vi "L2R.vi"() -> ()   [LabVIEW 2022 SP3]
uses:
  <vilib>/regexp/Match Regular Expression.xnode
panel:
  in  "SET_scale":dbl=1.0 caption="scaling:" min=0.01 max=200.0 step=0.1
  in  "SET_rotate":bool
  in  "SET_term_z_offs":dbl=20.0 caption="terminal z \noffset:"
  in  "SET_term_moc":u16(ring) caption="terminal\nmovement:" items=["NONE", "INSIDE", "-X", "-Y", "Z ONLY"]
  in  "SET_x_offs":dbl caption="X offset:"
  in  "SET_y_offs":dbl caption="Y offset:"
  out "OUT_choice":bool
  out "OUT_file_num":i32 caption="split files created"
  out "CONV_splitting":bool caption="FILE SPLITTING"
  out "OUT_comm_lines":i32 caption="command lines found"
  in  "SET_max_lines":i32=2000 caption="max. file lines"
  in  "SET_tool_angl":bool caption="tool \nangulation:"
  out "FILE_name_old":string caption="old\nfilename:"
  in  "FILE_name_new":string caption="new \nfilename:"
  in  "SET_zone":i32=10 caption="zone:"
  in  "SET_tool":string="tool0" caption="tool:"
  in  "SET_movtype":u16(ring) caption="movement \ntype:" items=["LINEAR", "JOINT"]
  out "ERR_write_file":errorcluster
  out "OUT_rapid":string caption="RAPID string"
  out "CONV_running":bool caption="CONVERSION RUNNING"
  out "ERR_read_file":errorcluster caption="read file error"
  in  "FILE_path":path caption="file path:\n(dialog)"
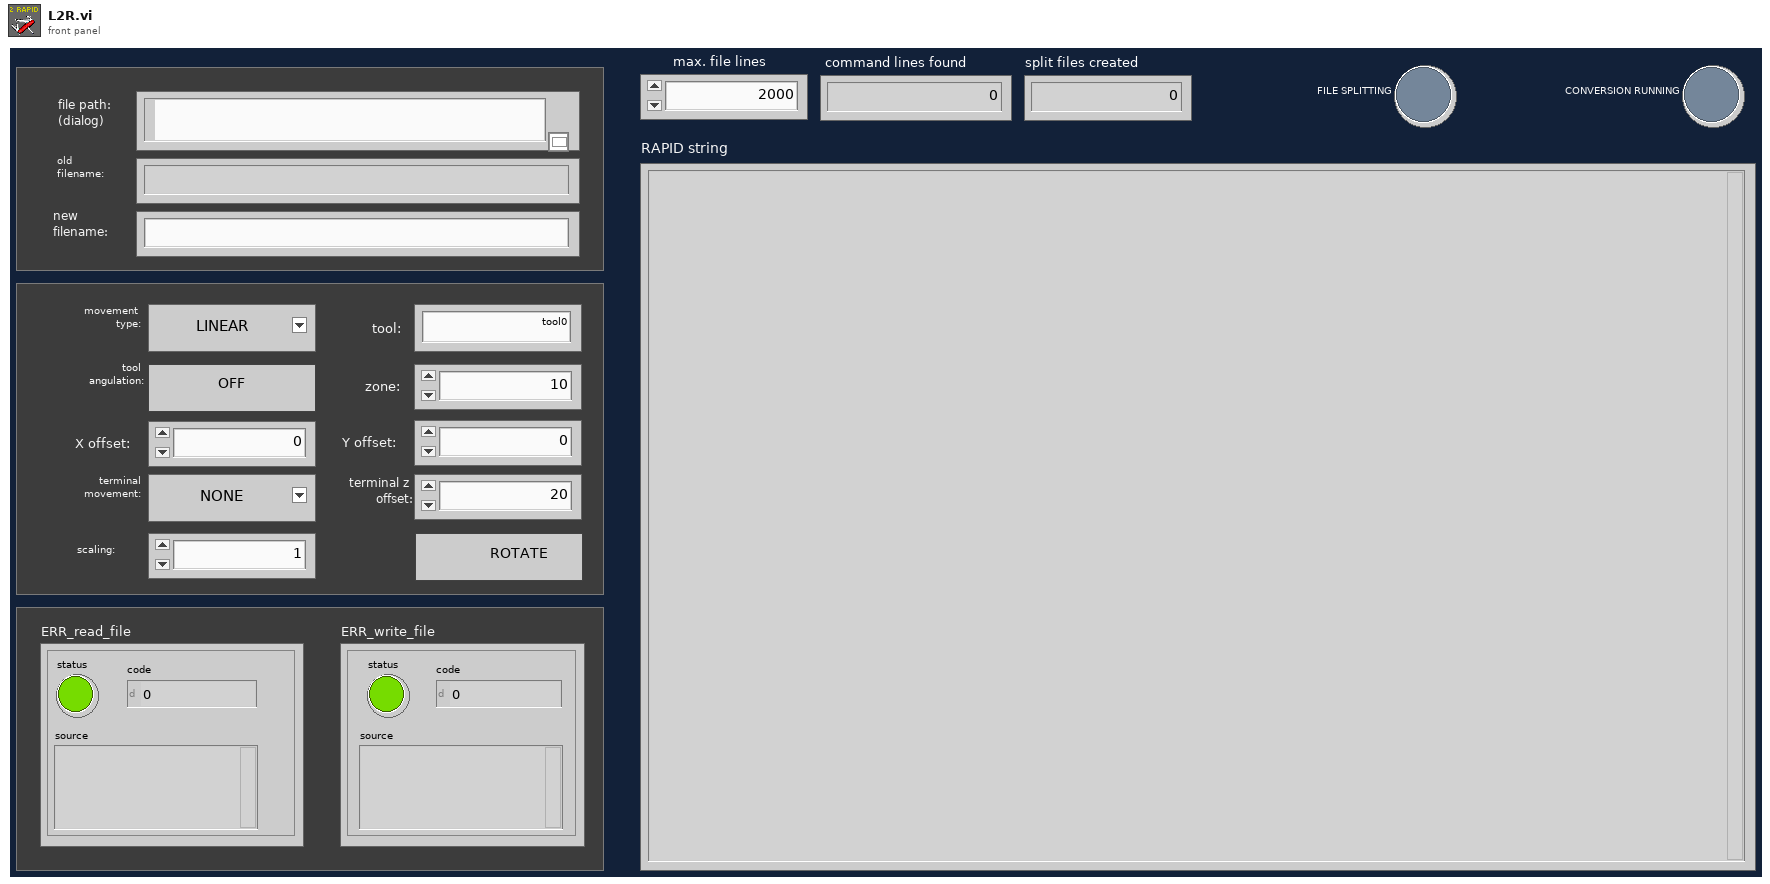
[diagram p1: front panel]
types:
  T1 = enum16{"open", "replace", "create", "open or create", "replace or create", "replace or create with confirmation"}
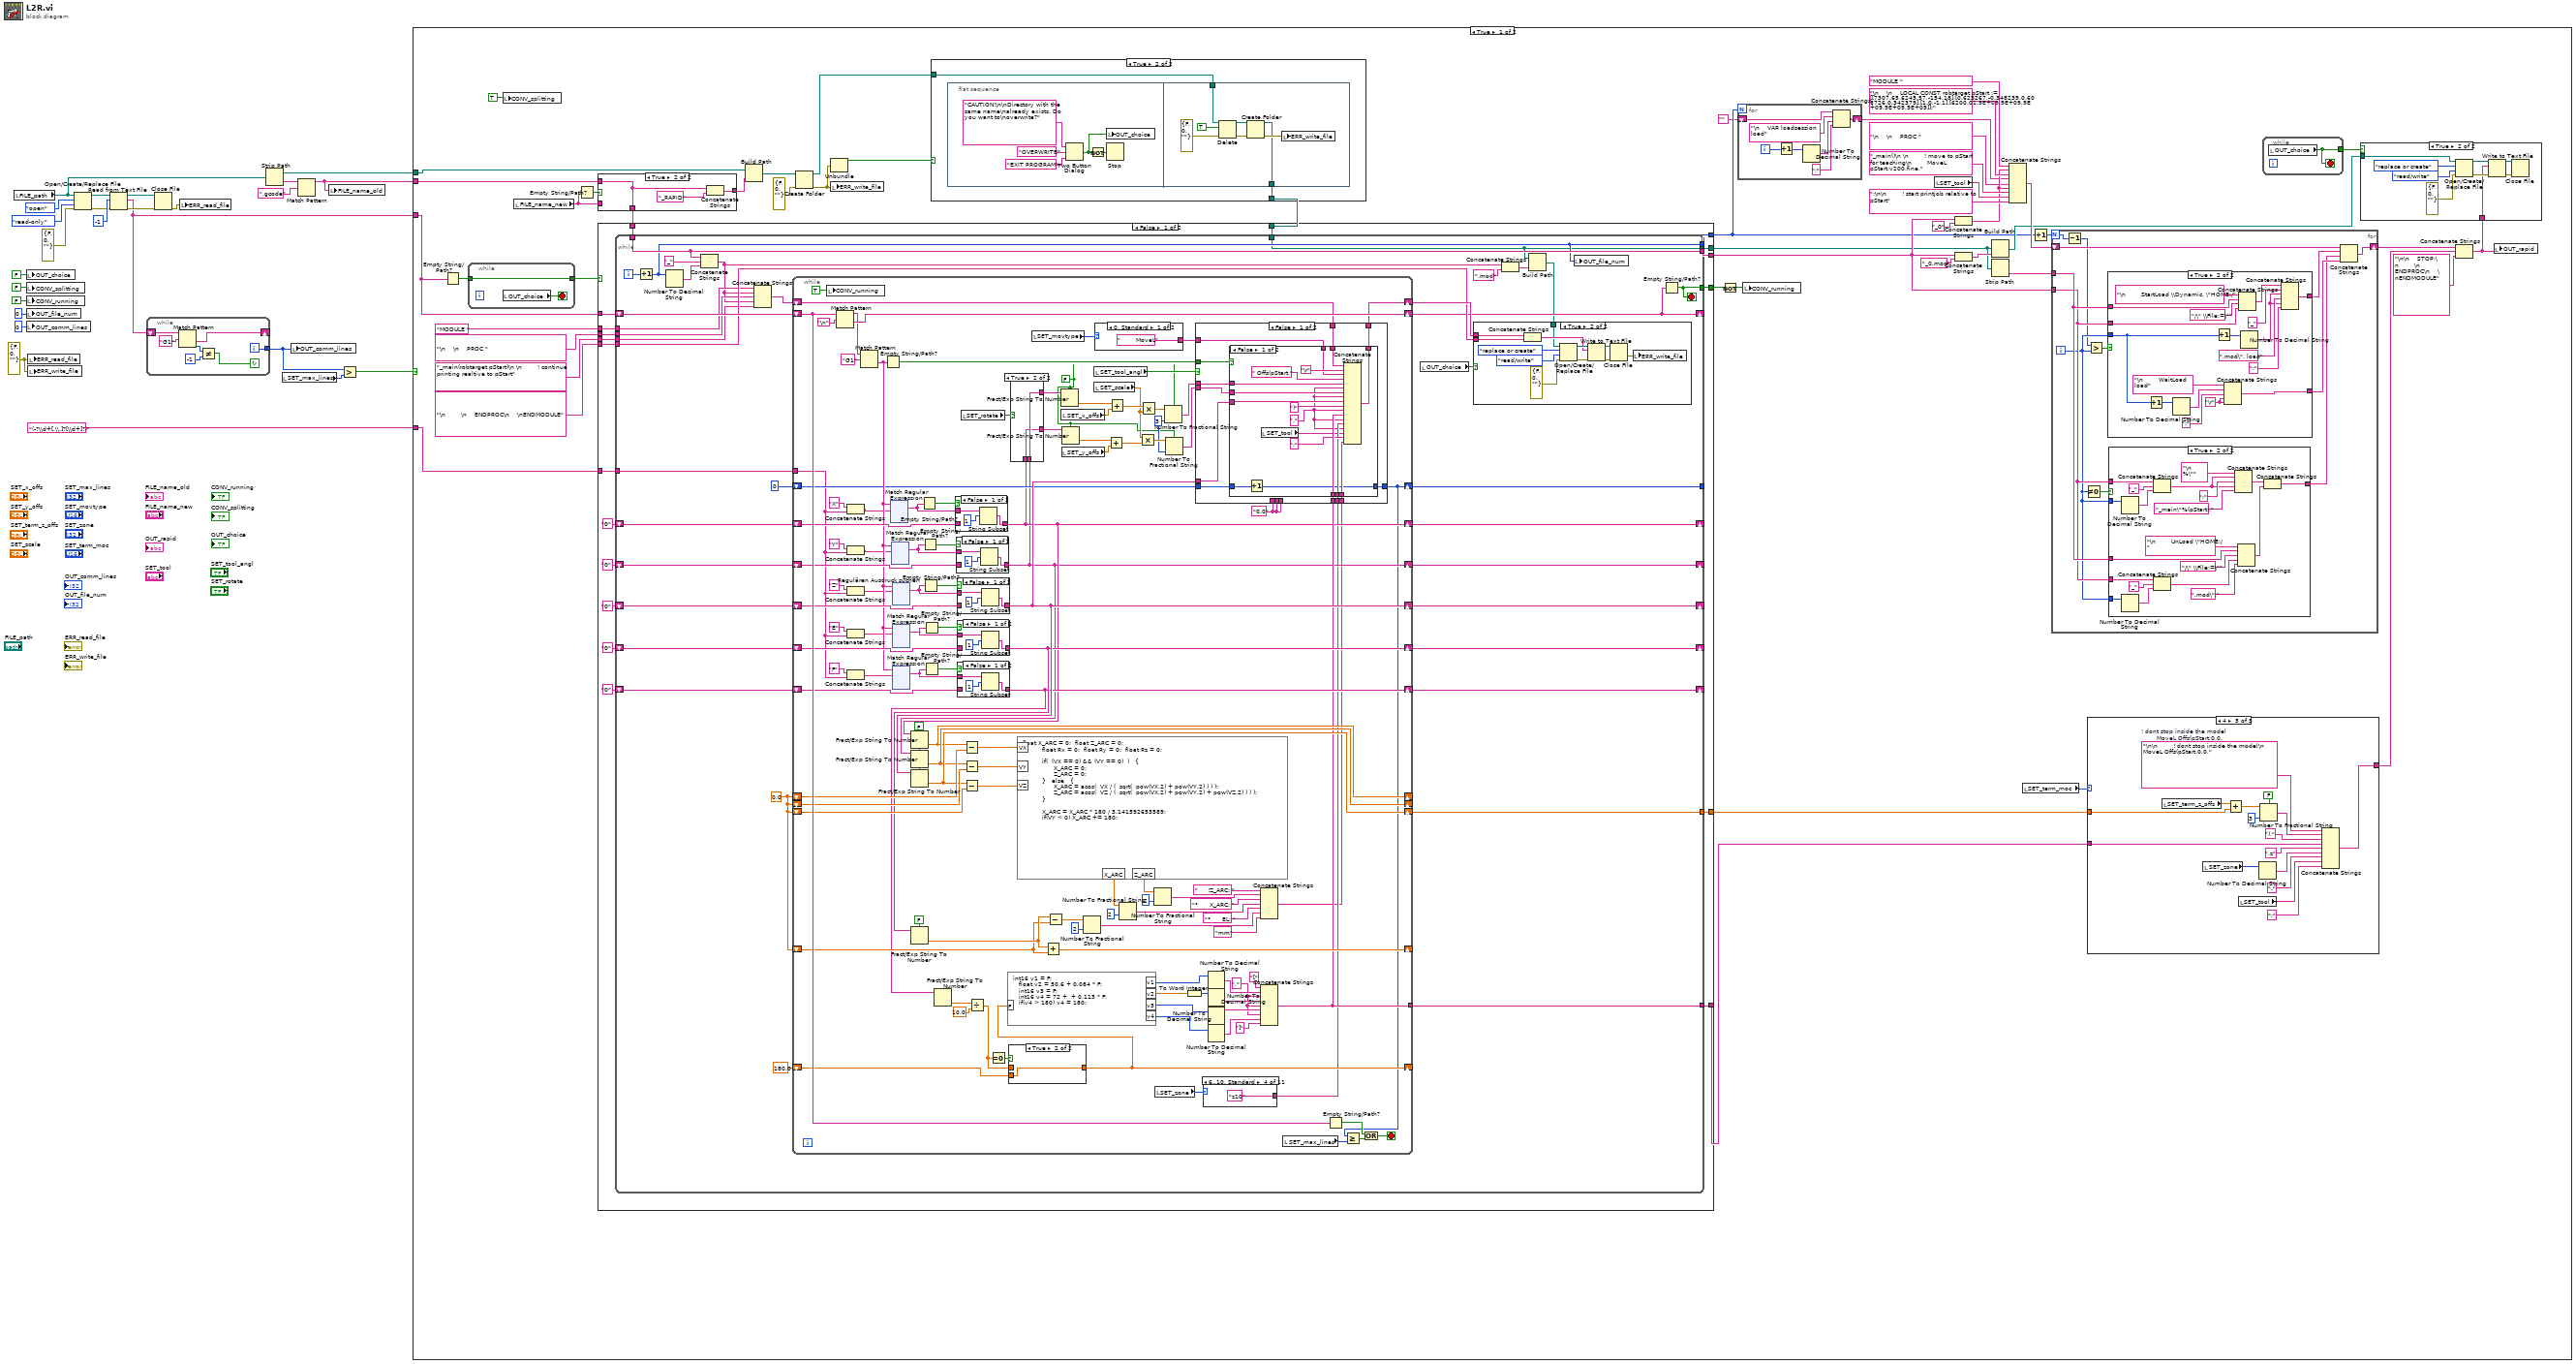
[diagram p0: block diagram]
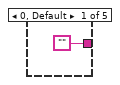
[diagram p2: hidden frame]
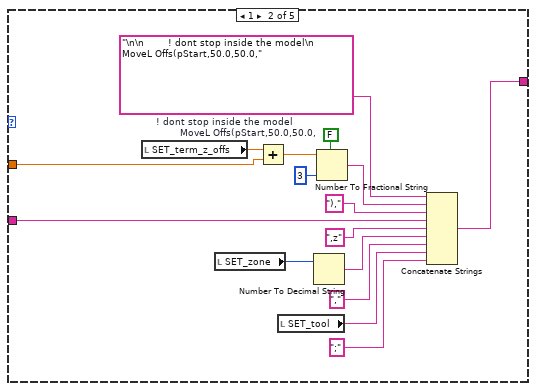
[diagram p3: hidden frame]
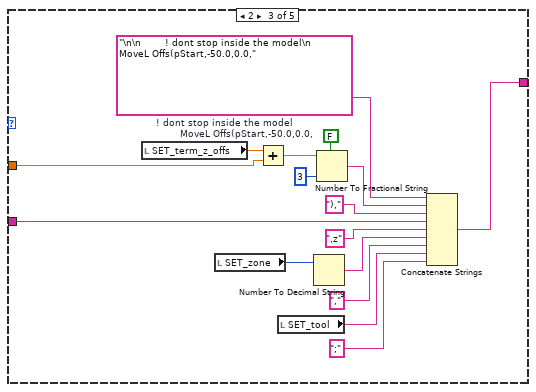
[diagram p4: hidden frame]
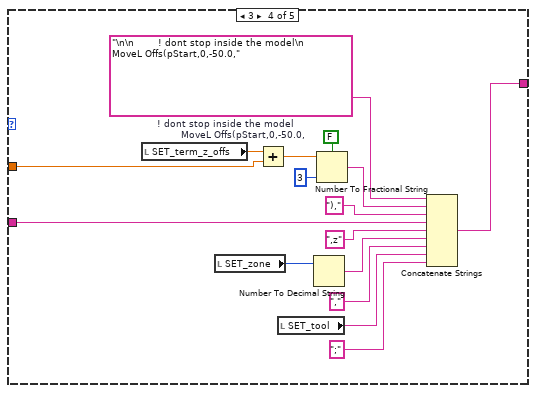
[diagram p5: hidden frame]
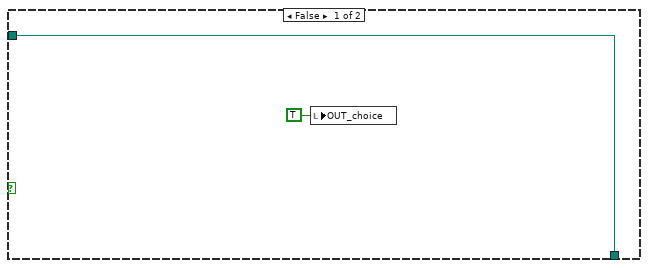
[diagram p7: hidden frame]
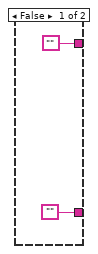
[diagram p8: hidden frame]
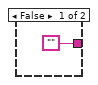
[diagram p9: hidden frame]
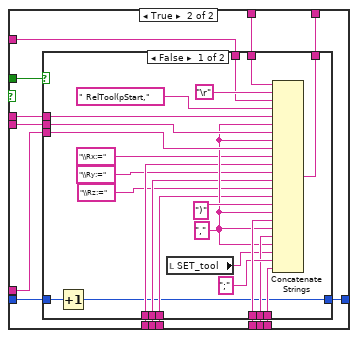
[diagram p15: hidden frame]
diagram:
  w6 = errorcluster {"status"=FALSE, "code"=0, "source"=""} ("ERR_write_file")
  n1 = local read "FILE_path"() -> (w10:path)
  n2 = local write "OUT_choice"(FALSE ("running")) -> ()
  n3 = local write "CONV_splitting"(FALSE ("running")) -> ()
  n4 = local write "CONV_running"(FALSE ("running")) -> ()
  n5 = local write "OUT_file_num"(0 ("OUT_file_num")) -> ()
  n6 = local write "OUT_comm_lines"(0 ("OUT_file_num")) -> ()
  n7 = local write "ERR_read_file"(w6) -> ()
  n8 = local write "ERR_write_file"(w6) -> ()
  n9 = Open/Create/Replace File(file path (use dialog)=w10, error in=errorcluster {"status"=FALSE, "code"=0, "source"=""}, operation (0:open)=T1."open", access (0:read/write)=enum16{"read/write", "read-only", "write-only"}."read-only") -> (refnum out=w21:refnum<file>, error out=w20:errorcluster)  [unwired: 2 in, 1 out]
  n10 = Read from Text File(file (use dialog)=w21, count=-1, error in=w20) -> (refnum out=w19:refnum<file>, text=w2:string, error out=w18:errorcluster)  [unwired: 1 in, 1 out]
  n11 = while {
    shift-right: [w30] -> _
    shift-left: w2 -> [w32]
    tunnel: [w26] -> w8
    i -> [w26]
    stop <- w27 continue-if-true
    n12 = Match Pattern(string=w32, regular expression="G1") -> (after substring=w30:string, offset past match=w29:i32)  [unwired: 1 in, 2 out]
    n13 = Not Equal?(x=w29, y=-1) -> (x != y?=w27:bool)
  }
  n14 = Close File(refnum=w19, error in=w18) -> (error out=w11:errorcluster)  [unwired: 1 out]
  n15 = local write "ERR_read_file"(w11) -> ()
  n16 = Strip Path(path=w10) -> (stripped path=w14:path, name=w16:string)
  n17 = local read "SET_max_lines"() -> (w12:i32)
  n18 = local write "OUT_comm_lines"(w8) -> ()
  n19 = Match Pattern(string=w16, regular expression=".gcode") -> (before substring=w9:string)  [unwired: 1 in, 3 out]
  n20 = local write "FILE_name_old"(w9) -> ()
  n21 = Greater?(x=w8, y=w12) -> (0:w13:bool)
  n22 = case shown="True" w13 {
    tunnel: w14 -> [w74 w1140]
    tunnel: w9 -> [w82 w1145]
    tunnel: w2 -> [w80 w1142]
    tunnel: "(-?\\d+[,\\.]?[\\d+]?)" ("regular expression") -> [w33 w1127]
    frame True {
      n23 = Empty String/Path?(string/path=w80) -> (empty?=w49:bool)
      n24 = while {
        tunnel: w49 -> [w156]
        tunnel: [w156] -> w48
        stop <- w157 stop-if-true
        n25 = local read "OUT_choice"() -> (w157:bool)
      }
      n26 = local write "CONV_splitting"(TRUE ("running")) -> ()
      n27 = local read "FILE_name_new"() -> (w79:string)
      n28 = Empty String/Path?(string/path=w79) -> (empty?=w81:bool)
      n29 = case shown="True" w81 {
        tunnel: w82 -> [_ w237]
        tunnel: w79 -> [w236 _]
        tunnel: [w236 w239] -> w72
        tunnel: [w236 w237] -> w76
        frame False {
        }
        frame True {
          n30 = Concatenate Strings(w237, "_RAPID" ("string")) -> (w239:string)
        }
      }
      n31 = Build Path(base path=w74, name or relative path=w72) -> (appended path=w73:path)
      n32 = Create Folder(path (use dialog)=w73, error in=errorcluster {"status"=FALSE, "code"=0, "source"=""}) -> (created path=w47:path, error out=w52:errorcluster)  [unwired: 1 in, 1 out]
      n33 = Unbundle(w52) -> ("status"=w51:bool)  [unwired: 2 out]
      n34 = local write "ERR_write_file"(w52) -> ()
      n35 = case shown="True" w51 {
        tunnel: w47 -> [w167 w170]
        tunnel: [w167 w169] -> w46
        frame False {
          n36 = local write "OUT_choice"(TRUE ("OUT_choice")) -> ()
        }
        frame True {
          n37 = flat-sequence {
            tunnel: w170 -> [w182]
            tunnel: [w176] -> w169
            frame #0 {
              n38 = Two Button Dialog(message="CAUTION!\n\nDirectory with the same name\nalready exists. Do you want to\noverwrite?", 1:"EXIT PROGRAM" ("F button name (\"Cancel\")"), 2:"OVERWRITE" ("T button name (\"OK\")")) -> (T button?=w171:bool)
              n39 = Not(x=w171) -> (.not. x?=w172:bool)
              n40 = Stop(stop? (T)=w172) -> ()
              n41 = local write "OUT_choice"(w171) -> ()
            }
            frame #1 {
              n42 = Delete(path (use dialog)=w182, entire hierarchy (F)=TRUE, error in=errorcluster {"status"=FALSE, "code"=0, "source"=""}) -> (deleted path=w180:path, error out=w179:errorcluster)  [unwired: 2 in, 1 out]
              n43 = Create Folder(path (use dialog)=w180, error in=w179) -> (created path=w176:path, error out=w177:errorcluster)  [unwired: 1 in, 1 out]
              n44 = local write "ERR_write_file"(w177) -> ()
            }
          }
        }
      }
      n45 = case shown="False" w48 {
        tunnel: w80 -> [w258 _]
        tunnel: "\n        \n    ENDPROC\n    \nENDMODULE" -> [w257 _]
        tunnel: [w256 FALSE] -> w77
        tunnel: w76 -> [w255 _]
        tunnel: "MODULE " -> [w254 _]
        tunnel: "\n    \n    PROC " -> [w253 _]
        tunnel: "_main(robtarget pStart)\n \n        ! continue printing realtive to pStart" -> [w252 _]
        tunnel: [w249 0 ("OUT_file_num")] -> w41
        tunnel: [w251 path "" ("created path")] -> w44
        tunnel: [w250 "" ("name")] -> w45
        tunnel: w46 -> [w248 _]
        tunnel: [w242 ""] -> w36
        tunnel: [w241 0.0] -> w37
        tunnel: w33 -> [w240 _]
        frame False {
          n46 = while {
            tunnel: w257 -> [w292]
            tunnel: [w291] -> w256
            tunnel: w255 -> [w278]
            tunnel: w254 -> [w290]
            tunnel: w253 -> [w289]
            tunnel: w252 -> [w288]
            shift-right: [w283] -> _
            shift-left: w258 -> [w295]
            tunnel: [w275] -> w251
            tunnel: [w278] -> w250
            tunnel: [w276] -> w249
            tunnel: w248 -> [w275]
            shift-right: [w268] -> _
            shift-left: "0" ("whole match") -> [w274]
            shift-right: [w267] -> _
            shift-left: "0" ("whole match") -> [w273]
            shift-right: [w266] -> _
            shift-left: "0" ("whole match") -> [w272]
            shift-right: [w265] -> _
            shift-left: "0" ("whole match") -> [w271]
            shift-right: [w264] -> _
            shift-left: "0" ("whole match") -> [w270]
            tunnel: [w269] -> _
            tunnel: [w261] -> w242
            tunnel: [w260] -> w241
            tunnel: w240 -> [w259]
            i -> [w286]
            stop <- w291 stop-if-true
            w262 = 0.0
            n47 = Increment(x=w286) -> (x+1=w276:i32)
            n48 = Number To Decimal String(number=w276) -> (decimal integer string=w284:string)  [unwired: 1 in]
            n49 = Concatenate Strings(w278, "_" ("string"), w284) -> (w281:string)
            n50 = Concatenate Strings(w290, w281, w289, w281, w288) -> (w287:string)
            n51 = while {
              shift-right: [w421] -> w283
              shift-left: w295 -> [w423]
              shift-right: [w417] -> w294
              shift-left: w287 -> [w418]
              shift-right: [w333] -> _
              shift-left: w262 -> [w401]
              shift-right: [w334] -> _
              shift-left: w262 -> [w400]
              shift-right: [w335] -> w260
              shift-left: w262 -> [w372]
              shift-right: [w331] -> w268
              shift-left: w274 -> [w394]
              shift-right: [w330] -> w267
              shift-left: w273 -> [w385]
              shift-right: [w381] -> w266
              shift-left: w272 -> [w384]
              shift-right: [w365] -> w265
              shift-left: w271 -> [w383]
              shift-right: [w356] -> w264
              shift-left: w270 -> [w382]
              shift-right: [w360] -> _
              shift-left: w262 -> [w358]
              shift-right: [w352] -> _
              shift-left: 180.0 -> [w353]
              shift-right: [w312] -> w269
              shift-left: 0 -> [w344]
              tunnel: [w332] -> w261
              tunnel: w259 -> [w313]
              stop <- w347 stop-if-true
              w309 = i16 3 ("Genauigkeit (6)")
              w308 = FALSE ("Systemdezimalzeichen verwenden (T)")
              w357 = "0.0"
              w377 = FALSE ("use system decimal point (T)")
              w404 = ","
              n52 = local write "CONV_running"(TRUE ("running")) -> ()
              n53 = Match Pattern(string=w423, regular expression="\n") -> (before substring=w420:string, after substring=w421:string)  [unwired: 1 in, 2 out]
              n54 = Concatenate Strings("X" ("regular expression"), w313) -> (w318:string)
              n55 = Concatenate Strings("Y" ("regular expression"), w313) -> (w317:string)
              n56 = Concatenate Strings("Z" ("regular expression"), w313) -> (w316:string)
              n57 = Concatenate Strings("E" ("regular expression"), w313) -> (w315:string)
              n58 = Concatenate Strings("F" ("regular expression"), w313) -> (w314:string)
              n59 = Match Pattern(string=w420, regular expression="G1") -> (after substring=w380:string)  [unwired: 1 in, 3 out]
              n60 = Empty String/Path?(string/path=w380) -> (empty?=w416:bool)
              n61 = xnode "Match Regular Expression"("input string"=w380, "regular expression"=w318) -> ("whole match"=w395:string)  [unwired: 4 in, 4 out]
              n62 = xnode "Match Regular Expression"("input string"=w380, "regular expression"=w317) -> ("whole match"=w393:string)  [unwired: 4 in, 4 out]
              n63 = xnode "Regulären Ausdruck suchen"("input string"=w380, "regular expression"=w316) -> ("whole match"=w390:string)  [unwired: 4 in, 4 out]
              n64 = xnode "Match Regular Expression"("input string"=w380, "regular expression"=w315) -> ("whole match"=w389:string)  [unwired: 4 in, 4 out]
              n65 = xnode "Match Regular Expression"("input string"=w380, "regular expression"=w314) -> ("whole match"=w386:string)  [unwired: 4 in, 4 out]
              n66 = Empty String/Path?(string/path=w395) -> (empty?=w396:bool)
              n67 = Empty String/Path?(string/path=w393) -> (empty?=w392:bool)
              n68 = Empty String/Path?(string/path=w390) -> (empty?=w391:bool)
              n69 = Empty String/Path?(string/path=w389) -> (empty?=w388:bool)
              n70 = Empty String/Path?(string/path=w386) -> (empty?=w387:bool)
              n71 = case shown="False" w396 {
                tunnel: w395 -> [w987 _]
                tunnel: [w985 w988] -> w331
                tunnel: w394 -> [_ w988]
                frame False {
                  n72 = String Subset(string=w987, offset (0)=1) -> (substring=w985:string)  [unwired: 1 in]
                }
                frame True {
                }
              }
              n73 = Fract/Exp String To Number(use system decimal point (T)=w377, string=w331) -> (number=w333:dbl)  [unwired: 2 in, 1 out]
              n74 = case shown="False" w392 {
                tunnel: w393 -> [w866 _]
                tunnel: [w864 w867] -> w330
                tunnel: w385 -> [_ w867]
                frame False {
                  n75 = String Subset(string=w866, offset (0)=1) -> (substring=w864:string)  [unwired: 1 in]
                }
                frame True {
                }
              }
              n76 = Fract/Exp String To Number(use system decimal point (T)=w377, string=w330) -> (number=w334:dbl)  [unwired: 2 in, 1 out]
              n77 = case shown="False" w391 {
                tunnel: w390 -> [w745 _]
                tunnel: [w743 w746] -> w381
                tunnel: w384 -> [_ w746]
                frame False {
                  n78 = String Subset(string=w745, offset (0)=1) -> (substring=w743:string)  [unwired: 1 in]
                }
                frame True {
                }
              }
              n79 = Fract/Exp String To Number(use system decimal point (T)=w377, string=w381) -> (number=w335:dbl)  [unwired: 2 in, 1 out]
              n80 = case shown="False" w388 {
                tunnel: w389 -> [w624 _]
                tunnel: [w622 w625] -> w365
                tunnel: w383 -> [_ w625]
                frame False {
                  n81 = String Subset(string=w624, offset (0)=1) -> (substring=w622:string)  [unwired: 1 in]
                }
                frame True {
                }
              }
              n82 = Fract/Exp String To Number(use system decimal point (T)=FALSE, string=w365) -> (number=w359:dbl)  [unwired: 2 in, 1 out]
              n83 = case shown="False" w387 {
                tunnel: w386 -> [w503 _]
                tunnel: [w501 w504] -> w356
                tunnel: w382 -> [_ w504]
                frame False {
                  n84 = String Subset(string=w503, offset (0)=1) -> (substring=w501:string)  [unwired: 1 in]
                }
                frame True {
                }
              }
              n85 = Fract/Exp String To Number(string=w356) -> (number=w379:dbl)  [unwired: 3 in, 1 out]
              n86 = local read "SET_rotate"() -> (w327:bool)
              n87 = Subtract(x=w333, y=w401) -> (x-y=w398:dbl)
              n88 = Subtract(x=w334, y=w400) -> (x-y=w399:dbl)
              n89 = Subtract(x=w335, y=w372) -> (x-y=w373:dbl)
              n90 = Divide(x=w379, y=10.0) -> (x/y=w354:dbl)
              n91 = Equal To 0?(x=w354) -> (x = 0?=w355:bool)
              n92 = case shown="True" w355 {
                tunnel: w354 -> [w428 _]
                tunnel: [w428 w429] -> w352
                tunnel: w353 -> [_ w429]
                frame False {
                }
                frame True {
                }
              }
              n93 = formula code="int16 v1 = F;\n   float v2 = 50.6 + 0.084 * F;\n   int16 v3 = F;\n   int16 v4 = 72 +  + 0.113 * F;\n   if(v4 > 180) v4 = 180;"("F"=w352) -> ("v1"=w413:i16, "v2"=w412:dbl, "v3"=w410:i16, "v4"=w409:i16)
              n94 = case shown="True" w327 {
                tunnel: w331 -> [w424 w426]
                tunnel: w330 -> [w425 w427]
                tunnel: [w425 w426] -> w329
                tunnel: [w424 w427] -> w328
                frame False {
                }
                frame True {
                }
              }
              n95 = formula code="float X_ARC = 0;  float Z_ARC = 0;\n          float Rx = 0;  float Ry = 0;  float Rz = 0;\n        \n          if(  (VX == 0) && (VY == 0)  )   {\n                X_ARC = 0;\n                Z_ARC = 0;\n          }   else   {\n                X_ARC = acos(  VX / (  sqrt(  pow(VX,2) + pow(VY,2) ) ) );\n                Z_ARC = acos(  VZ / (  sqrt(  pow(VX,2) + pow(VY,2) + pow(VZ,2) ) ) );\n          }\n        \n          X_ARC = X_ARC * 180 / 3.141592653589;\n          if(VY < 0) X_ARC += 180;"("VX"=w398, "VY"=w399, "VZ"=w373) -> ("X_ARC"=w371:dbl, "Z_ARC"=w369:dbl)
              n96 = local read "SET_movtype"() -> (w351:u16)
              n97 = Add(x=w359, y=w358) -> (x+y=w360:dbl)
              n98 = Subtract(x=w359, y=w358) -> (x-y=w361:dbl)
              n99 = Fract/Exp String To Number(use system decimal point (T)=w308, string=w328) -> (number=w343:dbl)  [unwired: 2 in, 1 out]
              n100 = local read "SET_x_offs"() -> (w341:dbl)
              n101 = Fract/Exp String To Number(use system decimal point (T)=w308, string=w329) -> (number=w337:dbl)  [unwired: 2 in, 1 out]
              n102 = local read "SET_y_offs"() -> (w339:dbl)
              n103 = Number To Fractional String(number=w361, precision (6)=i16 2) -> (F-format string=w362:string)  [unwired: 2 in]
              n104 = local read "SET_tool_angl"() -> (w349:bool)
              n105 = local read "SET_scale"() -> (w324:dbl)
              n106 = case shown="0, Standard" w351 {
                tunnel: ["        MoveL" "        MoveJ"] -> w415
                frame 0, Default {
                }
                frame 1 {
                }
              }
              n107 = Add(x=w337, y=w339) -> (x+y=w338:dbl)
              n108 = Add(x=w343, y=w341) -> (x+y=w342:dbl)
              n109 = Number To Fractional String(number=w371, precision (6)=i16 2) -> (F-format string=w367:string)  [unwired: 2 in]
              n110 = Multiply(x=w324, y=w338) -> (x*y=w325:dbl)
              n111 = Multiply(x=w342, y=w324) -> (x*y=w326:dbl)
              n112 = Number To Fractional String(number=w369, precision (6)=i16 2) -> (F-format string=w368:string)  [unwired: 2 in]
              n113 = local read "SET_zone"() -> (w348:i32)
              n114 = Number To Fractional String(use system decimal point (T)=w308, number=w326, precision (6)=w309) -> (F-format string=w340:string)  [unwired: 1 in]
              n115 = Number To Fractional String(use system decimal point (T)=w308, number=w325, precision (6)=w309) -> (F-format string=w336:string)  [unwired: 1 in]
              n116 = To Word Integer(number=w412) -> (16bit integer=w411:i16)
              n117 = case shown="6..10, Standard" w348 {
                tunnel: ["z1" "z2" "z5" "z10" "z20" "z50" "z100" "z200" "z300" "z400" "z500"] -> w311
                frame 0 {
                }
                frame 1, 2 {
                }
                frame 3..5 {
                }
                frame 6..10, Default {
                }
                frame 11..20 {
                }
                frame 21..50 {
                }
                frame 51..100 {
                }
                frame 101..200 {
                }
                frame 201..300 {
                }
                frame 301..400 {
                }
                frame 401..500 {
                }
              }
              n118 = Number To Decimal String(number=w413) -> (decimal integer string=w407:string)  [unwired: 1 in]
              n119 = Number To Decimal String(number=w411) -> (decimal integer string=w406:string)  [unwired: 1 in]
              n120 = Number To Decimal String(number=w410) -> (decimal integer string=w405:string)  [unwired: 1 in]
              n121 = Number To Decimal String(number=w409) -> (decimal integer string=w403:string)  [unwired: 1 in]
              n122 = Concatenate Strings("     !Z_ARC: ", w368, "°      X_ARC: ", w367, "°      EL: " ("string"), w362, "mm" ("string")) -> (w310:string)
              n123 = Concatenate Strings("[", w407, w404, w406, w404, w405, w404, w403, "]") -> (w332:string)
              n124 = case shown="False" w349 {
                tunnel: w418 -> [w441 w475]
                tunnel: [w440 w474] -> w417
                tunnel: w416 -> [w439 w473]
                tunnel: w415 -> [w438 w472]
                tunnel: w311 -> [w437 w471]
                tunnel: w332 -> [w436 w470]
                tunnel: w336 -> [w435 w469]
                tunnel: w340 -> [w434 w468]
                tunnel: w381 -> [w433 w467]
                tunnel: w310 -> [w432 w466]
                tunnel: w357 -> [_ w465]
                tunnel: w357 -> [_ w464]
                tunnel: w357 -> [_ w463]
                tunnel: [w430 w462] -> w312
                tunnel: w344 -> [w431 w461]
                frame False {
                  n125 = case shown="False" w439 {
                    tunnel: w441 -> [w458 w460]
                    tunnel: w434 -> [w455 _]
                    tunnel: w435 -> [w454 _]
                    tunnel: w433 -> [w453 _]
                    tunnel: w436 -> [w452 _]
                    tunnel: [w451 w460] -> w440
                    tunnel: w438 -> [w449 _]
                    tunnel: w437 -> [w447 _]
                    tunnel: w432 -> [w444 _]
                    tunnel: w431 -> [w443 w459]
                    tunnel: [w442 w459] -> w430
                    frame False {
                      w446 = ","
                      n126 = Increment(x=w443) -> (x+1=w442:i32)
                      n127 = local read "SET_tool"() -> (w445:string)
                      n128 = Concatenate Strings(w458, "\r", w449, " Offs(pStart,", w455, w446, w454, w446, w453, ")" ("string"), w446, w452, w446, w447, w446, w445, ";" ("string"), w444) -> (w451:string)
                    }
                    frame True {
                    }
                  }
                }
                frame True {
                  n129 = case shown="False" w473 {
                    tunnel: w475 -> [w498 w500]
                    tunnel: w468 -> [w495 _]
                    tunnel: w469 -> [w494 _]
                    tunnel: w467 -> [w493 _]
                    tunnel: w470 -> [w492 _]
                    tunnel: [w491 w500] -> w474
                    tunnel: w472 -> [w489 _]
                    tunnel: w471 -> [w487 _]
                    tunnel: w466 -> [w484 _]
                    tunnel: w465 -> [w483 _]
                    tunnel: w464 -> [w482 _]
                    tunnel: w463 -> [w481 _]
                    tunnel: [w477 w499] -> w462
                    tunnel: w461 -> [w476 w499]
                    frame False {
                      w486 = ","
                      n130 = Increment(x=w476) -> (x+1=w477:i32)
                      n131 = local read "SET_tool"() -> (w485:string)
                      n132 = Concatenate Strings(w498, "\r", w489, " RelTool(pStart,", w495, w486, w494, w486, w493, "\\Rx:=" ("string"), w483, "\\Ry:=" ("string"), w482, "\\Rz:=" ("string"), w481, ")" ("string"), w486, w492, w486, w487, w486, w485, ";" ("string"), w484) -> (w491:string)
                    }
                    frame True {
                    }
                  }
                }
              }
              n133 = local read "SET_max_lines"() -> (w345:i32)
              n134 = Empty String/Path?(string/path=w423) -> (empty?=w414:bool)
              n135 = Greater Or Equal?(x=w312, y=w345) -> (x >= y?=w346:bool)
              n136 = Or(x=w414, y=w346) -> (x .or. y?=w347:bool)
            }
            n137 = local read "OUT_choice"() -> (w277:bool)
            n138 = Concatenate Strings(w281, ".mod") -> (w280:string)
            n139 = Build Path(base path=w275, name or relative path=w280) -> (appended path=w279:path)
            n140 = case shown="True" w277 {
              tunnel: w294 -> [_ w307]
              tunnel: w292 -> [_ w306]
              tunnel: w279 -> [_ w296]
              frame False {
              }
              frame True {
                n141 = Concatenate Strings(w307, w306) -> (w297:string)
                n142 = Open/Create/Replace File(file path (use dialog)=w296, error in=errorcluster {"status"=FALSE, "code"=0, "source"=""}, operation (0:open)=T1."replace or create", access (0:read/write)=enum16{"read/write", "read-only", "write-only"}."read/write") -> (refnum out=w301:refnum<file>, error out=w302:errorcluster)  [unwired: 2 in, 1 out]
                n143 = Write to Text File(file (use dialog)=w301, text=w297, error in=w302) -> (refnum out=w303:refnum<file>, error out=w304:errorcluster)  [unwired: 1 in, 1 out]
                n144 = Close File(refnum=w303, error in=w304) -> (error out=w305:errorcluster)  [unwired: 1 out]
                n145 = local write "ERR_write_file"(w305) -> ()
              }
            }
            n146 = local write "OUT_file_num"(w276) -> ()
            n147 = Empty String/Path?(string/path=w283) -> (empty?=w291:bool)
          }
        }
        frame True {
          n148 = One Button Dialog(message="File is empty!", button name ("OK")="End program") -> ()  [unwired: 1 out]
        }
      }
      n149 = Not(x=w77) -> (.not. x?=w78:bool)
      n150 = for {
        N: w41 -> [_]
        shift-right: [w149] -> w39
        shift-left: "" -> [w148]
        i -> [w153]
        n151 = Increment(x=w153) -> (x+1=w154:i32)
        n152 = Number To Decimal String(number=w154) -> (decimal integer string=w151:string)  [unwired: 1 in]
        n153 = Concatenate Strings(w148, "\n    VAR loadsession load", w151, ";" ("string")) -> (w149:string)
      }
      n154 = local write "CONV_running"(w78) -> ()
      n155 = local read "SET_tool"() -> (w65:string)
      n156 = Concatenate Strings(w45, "_0" ("string")) -> (w63:string)
      n157 = Concatenate Strings(w45, "_0.mod" ("string")) -> (w69:string)
      n158 = Build Path(base path=w44, name or relative path=w69) -> (appended path=w60:path)
      n159 = Strip Path(path=w44) -> (name=w43:string)  [unwired: 1 out]
      n160 = Concatenate Strings("MODULE " ("string"), w63, "\n    \n    LOCAL CONST robtarget pStart := [[7307.65,6245.57,-154.18],[0.625267,-0.348239,0.608726,0.342379],[1,0,-1,1],[6200.01,9E+09,9E+09,9E+09,9E+09,9E+09]];" ("string"), w39, "\n    \n    PROC ", w63, "_main()\n \n        ! move to pStart for teaching\n        MoveL pStart,v200,fine," ("string"), w65, ";\n\n        ! start printjob relative to pStart" ("string")) -> (w61:string)
      n161 = local read "SET_term_moc"() -> (w34:u16)
      n162 = Increment(x=w41) -> (x+1=w42:i32)
      n163 = for {
        N: w42 -> [w190]
        shift-right: [w188] -> w59
        shift-left: w61 -> [w187]
        tunnel: w45 -> [w192]
        tunnel: w43 -> [w193]
        i -> [w189]
        n164 = Decrement(x=w190) -> (x-1=w183:i32)
        n165 = Not Equal To 0?(x=w189) -> (x != 0?=w194:bool)
        n166 = Greater?(x=w183, y=w189) -> (0:w191:bool)
        n167 = case shown="True" w191 {
          tunnel: w193 -> [_ w206]
          tunnel: w192 -> [_ w205]
          tunnel: w189 -> [_ w203]
          tunnel: ["" w199] -> w185
          tunnel: ["" w198] -> w186
          frame False {
          }
          frame True {
            w197 = "\r"
            n168 = Increment(x=w203) -> (x+1=w204:i32)
            n169 = Number To Decimal String(number=w204) -> (decimal integer string=w201:string)  [unwired: 1 in]
            n170 = Increment(x=w203) -> (x+1=w212:i32)
            n171 = Concatenate Strings("\n        WaitLoad load", w201, ";" ("string"), w197, w197) -> (w199:string)
            n172 = Concatenate Strings("\n        StartLoad \\Dynamic, \"HOME:/", w206, "/\" \\File:=\"" ("String"), w205) -> (w207:string)
            n173 = Number To Decimal String(number=w212) -> (decimal integer string=w211:string)  [unwired: 1 in]
            n174 = Concatenate Strings(w207, "_" ("string"), w211, ".mod\", load" ("string"), w211, ";") -> (w198:string)
          }
        }
        n175 = case shown="True" w194 {
          tunnel: w189 -> [_ w228]
          tunnel: w192 -> [_ w234]
          tunnel: w193 -> [_ w226]
          tunnel: w192 -> [_ w223]
          tunnel: w189 -> [_ w222]
          tunnel: ["" w217] -> w184
          frame False {
          }
          frame True {
            n176 = Number To Decimal String(number=w228) -> (decimal integer string=w232:string)  [unwired: 1 in]
            n177 = Number To Decimal String(number=w222) -> (decimal integer string=w221:string)  [unwired: 1 in]
            n178 = Concatenate Strings(w234, "_" ("string"), w232) -> (w230:string)
            n179 = Concatenate Strings(w223, "_" ("string"), w221) -> (w220:string)
            n180 = Concatenate Strings("\n        %\"", w230, ":", w230, "_main\"%(pStart);" ("String")) -> (w219:string)
            n181 = Concatenate Strings("\n        UnLoad \"HOME:/", w226, "/\" \\File:=\"" ("String"), w220, ".mod\";" ("string")) -> (w218:string)
            n182 = Concatenate Strings(w219, w218) -> (w217:string)
          }
        }
        n183 = Concatenate Strings(w187, w186, w184, w185) -> (w188:string)
      }
      n184 = case shown="4" w34 {
        tunnel: ["" w99 w100 w117 w134] -> w35
        tunnel: w36 -> [_ w96 w102 w119 w133]
        tunnel: w37 -> [_ w94 w106 w116 w132]
        frame 0, Default {
        }
        frame 1 {
          w98 = "\n\n        ! dont stop inside the model\n        MoveL Offs(pStart,50.0,50.0,"  # ! dont stop inside the model         MoveL Offs(pStart,50.0,50.0,
          n185 = local read "SET_term_z_offs"() -> (w90:dbl)
          n186 = local read "SET_zone"() -> (w87:i32)
          n187 = Add(x=w90, y=w94) -> (x+y=w91:dbl)
          n188 = local read "SET_tool"() -> (w85:string)
          n189 = Number To Decimal String(number=w87) -> (decimal integer string=w86:string)  [unwired: 1 in]
          n190 = Number To Fractional String(use system decimal point (T)=FALSE ("Systemdezimalzeichen verwenden (T)"), number=w91, precision (6)=i16 3 ("Genauigkeit (6)")) -> (F-format string=w92:string)  [unwired: 1 in]
          n191 = Concatenate Strings(w98, w92, "),", w96, ",z", w86, "," ("String"), w85, ";" ("String")) -> (w99:string)
        }
        frame 2 {
          w101 = "\n\n        ! dont stop inside the model\n        MoveL Offs(pStart,-50.0,0.0,"  # ! dont stop inside the model         MoveL Offs(pStart,-50.0,0.0,
          n192 = local read "SET_term_z_offs"() -> (w105:dbl)
          n193 = local read "SET_zone"() -> (w104:i32)
          n194 = Add(x=w105, y=w106) -> (x+y=w114:dbl)
          n195 = local read "SET_tool"() -> (w103:string)
          n196 = Number To Decimal String(number=w104) -> (decimal integer string=w115:string)  [unwired: 1 in]
          n197 = Number To Fractional String(use system decimal point (T)=FALSE ("Systemdezimalzeichen verwenden (T)"), number=w114, precision (6)=i16 3 ("Genauigkeit (6)")) -> (F-format string=w113:string)  [unwired: 1 in]
          n198 = Concatenate Strings(w101, w113, "),", w102, ",z", w115, "," ("String"), w103, ";" ("String")) -> (w100:string)
        }
        frame 3 {
          w118 = "\n\n        ! dont stop inside the model\n        MoveL Offs(pStart,0,-50.0,"  # ! dont stop inside the model         MoveL Offs(pStart,0,-50.0,
          n199 = local read "SET_term_z_offs"() -> (w128:dbl)
          n200 = local read "SET_zone"() -> (w127:i32)
          n201 = Add(x=w128, y=w116) -> (x+y=w130:dbl)
          n202 = local read "SET_tool"() -> (w126:string)
          n203 = Number To Decimal String(number=w127) -> (decimal integer string=w131:string)  [unwired: 1 in]
          n204 = Number To Fractional String(use system decimal point (T)=FALSE ("Systemdezimalzeichen verwenden (T)"), number=w130, precision (6)=i16 3 ("Genauigkeit (6)")) -> (F-format string=w129:string)  [unwired: 1 in]
          n205 = Concatenate Strings(w118, w129, "),", w119, ",z", w131, "," ("String"), w126, ";" ("String")) -> (w117:string)
        }
        frame 4 {
          w135 = "\n\n        ! dont stop inside the model\n        MoveL Offs(pStart,0,0,"  # ! dont stop inside the model         MoveL Offs(pStart,0,0,
          n206 = local read "SET_term_z_offs"() -> (w144:dbl)
          n207 = local read "SET_zone"() -> (w143:i32)
          n208 = Add(x=w144, y=w132) -> (x+y=w146:dbl)
          n209 = local read "SET_tool"() -> (w142:string)
          n210 = Number To Decimal String(number=w143) -> (decimal integer string=w147:string)  [unwired: 1 in]
          n211 = Number To Fractional String(use system decimal point (T)=FALSE ("Systemdezimalzeichen verwenden (T)"), number=w146, precision (6)=i16 3 ("Genauigkeit (6)")) -> (F-format string=w145:string)  [unwired: 1 in]
          n212 = Concatenate Strings(w135, w145, "),", w133, ",z", w147, "," ("String"), w142, ";" ("String")) -> (w134:string)
        }
      }
      n213 = while {
        tunnel: [w155] -> w50
        stop <- w155 stop-if-true
        n214 = local read "OUT_choice"() -> (w155:bool)
      }
      n215 = Concatenate Strings(w59, w35, "\n\n    STOP;\n        \n    ENDPROC\n    \nENDMODULE" ("string")) -> (w57:string)
      n216 = case shown="True" w50 {
        tunnel: w60 -> [_ w160]
        tunnel: w57 -> [_ w159]
        frame False {
        }
        frame True {
          n217 = Open/Create/Replace File(file path (use dialog)=w160, error in=errorcluster {"status"=FALSE, "code"=0, "source"=""}, operation (0:open)=T1."replace or create", access (0:read/write)=enum16{"read/write", "read-only", "write-only"}."read/write") -> (refnum out=w163:refnum<file>, error out=w164:errorcluster)  [unwired: 2 in, 1 out]
          n218 = Write to Text File(file (use dialog)=w163, text=w159, error in=w164) -> (refnum out=w165:refnum<file>, error out=w166:errorcluster)  [unwired: 1 in, 1 out]
          n219 = Close File(refnum=w165, error in=w166) -> ()  [unwired: 2 out]
        }
      }
      n220 = local write "OUT_rapid"(w57) -> ()
    }
    frame False {
      n221 = local read "SET_tool"() -> (w1135:string)
      n222 = local read "FILE_name_new"() -> (w1141:string)
      n223 = Empty String/Path?(string/path=w1141) -> (empty?=w1144:bool)
      n224 = case shown="True" w1144 {
        tunnel: w1145 -> [_ w1177]
        tunnel: w1141 -> [w1176 _]
        tunnel: [w1175 w1179] -> w1139
        tunnel: [w1176 w1177] -> w1143
        frame False {
          n225 = Concatenate Strings(w1176, ".mod" ("string")) -> (w1175:string)
        }
        frame True {
          n226 = Concatenate Strings(w1177, "_RAPID.mod" ("string")) -> (w1179:string)
        }
      }
      n227 = Concatenate Strings("MODULE ", w1143, "\n    \n    LOCAL CONST robtarget pStart := [[7307.65,6245.57,-154.18],[0.625267,-0.348239,0.608726,0.342379],[1,0,-1,1],[6200.01,9E+09,9E+09,9E+09,9E+09,9E+09]];\n    \n    PROC ", w1143, "_main()\n \n        ! move to pStart for teaching\n        MoveL pStart,v200,fine,", w1135, ";\n\n        ! start printjob relative to pStart" ("string")) -> (w1146:string)
      n228 = Empty String/Path?(string/path=w1142) -> (empty?=w1150:bool)
      n229 = case shown="False" w1150 {
        tunnel: w1142 -> [w1199 _]
        tunnel: w1146 -> [w1198 _]
        tunnel: [w1197 w2057] -> w1131
        tunnel: "       \n    ENDPROC\n    \nENDMODULE" -> [w1186 _]
        tunnel: w1127 -> [w1180 _]
        frame False {
          w1188 = 0.0
          n230 = while {
            shift-right: [w1369] -> _
            shift-left: w1199 -> [w1371]
            shift-right: [w1365] -> w1196
            shift-left: w1198 -> [w1366]
            tunnel: [w1362] -> w1195
            shift-right: [w1349] -> _
            shift-left: w1188 -> [w1347]
            shift-right: [w1348] -> _
            shift-left: w1188 -> [w1346]
            shift-right: [w1320] -> _
            shift-left: w1188 -> [w1318]
            shift-right: [w1278] -> _
            shift-left: "0" ("whole match") -> [w1340]
            shift-right: [w1277] -> _
            shift-left: "0" ("whole match") -> [w1331]
            shift-right: [w1282] -> _
            shift-left: "0" ("whole match") -> [w1330]
            shift-right: [w1310] -> _
            shift-left: "0" ("whole match") -> [w1329]
            shift-right: [w1301] -> _
            shift-left: "0" ("whole match") -> [w1328]
            shift-right: [w1305] -> _
            shift-left: 0.0 -> [w1303]
            shift-right: [w1297] -> _
            shift-left: 180.0 -> [w1298]
            tunnel: [w1284] -> w1182
            tunnel: [w1281] -> w1183
            tunnel: w1180 -> [w1260]
            stop <- w1362 stop-if-true
            w1258 = i16 3 ("Genauigkeit (6)")
            w1257 = FALSE ("Systemdezimalzeichen verwenden (T)")
            w1302 = "0.0"
            w1324 = FALSE ("use system decimal point (T)")
            w1352 = ","
            n231 = local write "CONV_running"(TRUE ("running")) -> ()
            n232 = Match Pattern(string=w1371, regular expression="\n") -> (before substring=w1368:string, after substring=w1369:string)  [unwired: 1 in, 2 out]
            n233 = Concatenate Strings("X" ("regular expression"), w1260) -> (w1270:string)
            n234 = Concatenate Strings("Y" ("regular expression"), w1260) -> (w1267:string)
            n235 = Concatenate Strings("Z" ("regular expression"), w1260) -> (w1265:string)
            n236 = Concatenate Strings("E" ("regular expression"), w1260) -> (w1263:string)
            n237 = Concatenate Strings("F" ("regular expression"), w1260) -> (w1261:string)
            n238 = Match Pattern(string=w1368, regular expression="G1") -> (after substring=w1327:string)  [unwired: 1 in, 3 out]
            n239 = Empty String/Path?(string/path=w1327) -> (empty?=w1364:bool)
            n240 = xnode "Regulären Ausdruck suchen"("input string"=w1327, "regular expression"=w1270) -> ("whole match"=w1341:string)  [unwired: 4 in, 4 out]
            n241 = xnode "Match Regular Expression"("input string"=w1327, "regular expression"=w1267) -> ("whole match"=w1339:string)  [unwired: 4 in, 4 out]
            n242 = xnode "Match Regular Expression"("input string"=w1327, "regular expression"=w1265) -> ("whole match"=w1336:string)  [unwired: 4 in, 4 out]
            n243 = xnode "Match Regular Expression"("input string"=w1327, "regular expression"=w1263) -> ("whole match"=w1335:string)  [unwired: 4 in, 4 out]
            n244 = xnode "Match Regular Expression"("input string"=w1327, "regular expression"=w1261) -> ("whole match"=w1332:string)  [unwired: 4 in, 4 out]
            n245 = Empty String/Path?(string/path=w1341) -> (empty?=w1342:bool)
            n246 = Empty String/Path?(string/path=w1339) -> (empty?=w1338:bool)
            n247 = Empty String/Path?(string/path=w1336) -> (empty?=w1337:bool)
            n248 = Empty String/Path?(string/path=w1335) -> (empty?=w1334:bool)
            n249 = Empty String/Path?(string/path=w1332) -> (empty?=w1333:bool)
            n250 = local read "SET_movtype"() -> (w1296:u16)
            n251 = case shown="False" w1342 {
              tunnel: w1341 -> [w1924 _]
              tunnel: [w1923 w1926] -> w1278
              tunnel: w1340 -> [_ w1926]
              frame False {
                n252 = String Subset(string=w1924, offset (0)=1) -> (substring=w1923:string)  [unwired: 1 in]
              }
              frame True {
              }
            }
            n253 = Fract/Exp String To Number(use system decimal point (T)=w1324, string=w1278) -> (number=w1349:dbl)  [unwired: 2 in, 1 out]
            n254 = case shown="False" w1338 {
              tunnel: w1339 -> [w1803 _]
              tunnel: [w1802 w1805] -> w1277
              tunnel: w1331 -> [_ w1805]
              frame False {
                n255 = String Subset(string=w1803, offset (0)=1) -> (substring=w1802:string)  [unwired: 1 in]
              }
              frame True {
              }
            }
            n256 = Fract/Exp String To Number(use system decimal point (T)=w1324, string=w1277) -> (number=w1348:dbl)  [unwired: 2 in, 1 out]
            n257 = case shown="False" w1337 {
              tunnel: w1336 -> [w1682 _]
              tunnel: [w1681 w1684] -> w1282
              tunnel: w1330 -> [_ w1684]
              frame False {
                n258 = String Subset(string=w1682, offset (0)=1) -> (substring=w1681:string)  [unwired: 1 in]
              }
              frame True {
              }
            }
            n259 = Fract/Exp String To Number(use system decimal point (T)=w1324, string=w1282) -> (number=w1320:dbl)  [unwired: 2 in, 1 out]
            n260 = case shown="False" w1334 {
              tunnel: w1335 -> [w1561 _]
              tunnel: [w1560 w1563] -> w1310
              tunnel: w1329 -> [_ w1563]
              frame False {
                n261 = String Subset(string=w1561, offset (0)=1) -> (substring=w1560:string)  [unwired: 1 in]
              }
              frame True {
              }
            }
            n262 = Fract/Exp String To Number(use system decimal point (T)=FALSE, string=w1310) -> (number=w1304:dbl)  [unwired: 2 in, 1 out]
            n263 = case shown="False" w1333 {
              tunnel: w1332 -> [w1441 _]
              tunnel: [w1439 w1442] -> w1301
              tunnel: w1328 -> [_ w1442]
              frame False {
                n264 = String Subset(string=w1441, offset (0)=1) -> (substring=w1439:string)  [unwired: 1 in]
              }
              frame True {
              }
            }
            n265 = Fract/Exp String To Number(use system decimal point (T)=FALSE ("Systemdezimalzeichen verwenden (T)"), string=w1301) -> (number=w1326:dbl)  [unwired: 2 in, 1 out]
            n266 = local read "SET_rotate"() -> (w1274:bool)
            n267 = Subtract(x=w1349, y=w1347) -> (x-y=w1344:dbl)
            n268 = Subtract(x=w1348, y=w1346) -> (x-y=w1345:dbl)
            n269 = Subtract(x=w1320, y=w1318) -> (x-y=w1319:dbl)
            n270 = Subtract(x=w1304, y=w1303) -> (x-y=w1306:dbl)
            n271 = Add(x=w1304, y=w1303) -> (x+y=w1305:dbl)
            n272 = Divide(x=w1326, y=10.0) -> (x/y=w1299:dbl)
            n273 = Equal To 0?(x=w1299) -> (x = 0?=w1300:bool)
            n274 = Absolute Value(x=w1306) -> (abs(x)=w1280:dbl)
            n275 = case shown="False" w1300 {
              tunnel: w1299 -> [w1376 _]
              tunnel: [w1376 w1377] -> w1297
              tunnel: w1298 -> [_ w1377]
              frame False {
              }
              frame True {
              }
            }
            n276 = formula code="int16 v1 = F;\n   float v2 = 50.6 + 0.084 * F;\n   int16 v3 = F;\n   int16 v4 = 72 +  + 0.113 * F;\n   if(v4 > 180) v4 = 180;"("F"=w1297) -> ("v1"=w1361:i16, "v2"=w1360:dbl, "v3"=w1358:i16, "v4"=w1357:i16)
            n277 = case shown="True" w1274 {
              tunnel: w1278 -> [w1372 w1374]
              tunnel: w1277 -> [w1373 w1375]
              tunnel: [w1373 w1374] -> w1276
              tunnel: [w1372 w1375] -> w1275
              frame False {
              }
              frame True {
              }
            }
            n278 = formula code="float X_ARC = 0;  float Z_ARC = 0;\n          float Rx = 0;  float Ry = 0;  float Rz = 0;\n        \n          if(  (VX == 0) && (VY == 0)  )   {\n                X_ARC = 0;\n                Z_ARC = 0;\n          }   else   {\n                X_ARC = acos(  VX / (  sqrt(  pow(VX,2) + pow(VY,2) ) ) );\n                Z_ARC = acos(  VZ / (  sqrt(  pow(VX,2) + pow(VY,2) + pow(VZ,2) ) ) );\n          }\n        \n          X_ARC = X_ARC * 180 / 3.141592653589;\n          if(VY < 0) X_ARC += 180;"("VX"=w1344, "VY"=w1345, "VZ"=w1319) -> ("X_ARC"=w1317:dbl, "Z_ARC"=w1315:dbl)
            n279 = case shown="0, Standard" w1296 {
              tunnel: ["        MoveL" "        MoveJ"] -> w1363
              frame 0, Default {
              }
              frame 1 {
              }
            }
            n280 = Number To Fractional String(number=w1280, precision (6)=i16 2) -> (F-format string=w1307:string)  [unwired: 2 in]
            n281 = Fract/Exp String To Number(use system decimal point (T)=w1257, string=w1275) -> (number=w1292:dbl)  [unwired: 2 in, 1 out]
            n282 = Fract/Exp String To Number(use system decimal point (T)=w1257, string=w1276) -> (number=w1287:dbl)  [unwired: 2 in, 1 out]
            n283 = local read "SET_tool_angl"() -> (w1294:bool)
            n284 = local read "SET_x_offs"() -> (w1290:dbl)
            n285 = local read "SET_y_offs"() -> (w1289:dbl)
            n286 = local read "SET_scale"() -> (w1271:dbl)
            n287 = Number To Fractional String(number=w1317, precision (6)=i16 2) -> (F-format string=w1313:string)  [unwired: 2 in]
            n288 = Add(x=w1292, y=w1290) -> (x+y=w1291:dbl)
            n289 = Add(x=w1287, y=w1289) -> (x+y=w1288:dbl)
            n290 = Number To Fractional String(number=w1315, precision (6)=i16 2) -> (F-format string=w1314:string)  [unwired: 2 in]
            n291 = local read "SET_zone"() -> (w1293:i32)
            n292 = Multiply(x=w1288, y=w1271) -> (x*y=w1272:dbl)
            n293 = Multiply(x=w1291, y=w1271) -> (x*y=w1273:dbl)
            n294 = To Word Integer(number=w1360) -> (16bit integer=w1359:i16)
            n295 = Number To Fractional String(use system decimal point (T)=w1257, number=w1273, precision (6)=w1258) -> (F-format string=w1286:string)  [unwired: 1 in]
            n296 = Number To Fractional String(use system decimal point (T)=w1257, number=w1272, precision (6)=w1258) -> (F-format string=w1285:string)  [unwired: 1 in]
            n297 = case shown="0" w1293 {
              tunnel: ["z1" "z2" "z5" "z10" "z20" "z50" "z100" "z200" "z300" "z400" "z500"] -> w1259
              frame 0 {
              }
              frame 1, 2 {
              }
              frame 3..5 {
              }
              frame 6..10, Default {
              }
              frame 11..20 {
              }
              frame 21..50 {
              }
              frame 51..100 {
              }
              frame 101..200 {
              }
              frame 201..300 {
              }
              frame 301..400 {
              }
              frame 401..500 {
              }
            }
            n298 = Number To Decimal String(number=w1361) -> (decimal integer string=w1355:string)  [unwired: 1 in]
            n299 = Number To Decimal String(number=w1359) -> (decimal integer string=w1354:string)  [unwired: 1 in]
            n300 = Number To Decimal String(number=w1358) -> (decimal integer string=w1353:string)  [unwired: 1 in]
            n301 = Number To Decimal String(number=w1357) -> (decimal integer string=w1351:string)  [unwired: 1 in]
            n302 = Concatenate Strings("     !Z_ARC: ", w1314, "°      X_ARC: ", w1313, "°      EL: " ("string"), w1307, "mm" ("string")) -> (w1311:string)
            n303 = Concatenate Strings("[", w1355, w1352, w1354, w1352, w1353, w1352, w1351, "]") -> (w1284:string)
            n304 = case shown="True" w1294 {
              tunnel: w1366 -> [w1387 w1416]
              tunnel: [w1386 w1415] -> w1365
              tunnel: w1364 -> [w1385 w1414]
              tunnel: w1363 -> [w1384 w1413]
              tunnel: w1259 -> [w1383 w1412]
              tunnel: w1284 -> [w1382 w1411]
              tunnel: w1285 -> [w1381 w1410]
              tunnel: w1286 -> [w1380 w1409]
              tunnel: w1282 -> [w1379 w1408]
              tunnel: w1311 -> [w1378 w1407]
              tunnel: w1302 -> [_ w1406]
              tunnel: w1302 -> [_ w1405]
              tunnel: w1302 -> [_ w1404]
              frame False {
                n305 = case shown="False" w1385 {
                  tunnel: w1387 -> [w1402 w1403]
                  tunnel: w1380 -> [w1399 _]
                  tunnel: w1381 -> [w1398 _]
                  tunnel: w1379 -> [w1397 _]
                  tunnel: w1382 -> [w1396 _]
                  tunnel: [w1395 w1403] -> w1386
                  tunnel: w1384 -> [w1393 _]
                  tunnel: w1383 -> [w1391 _]
                  tunnel: w1378 -> [w1388 _]
                  frame False {
                    w1390 = ","
                    n306 = local read "SET_tool"() -> (w1389:string)
                    n307 = Concatenate Strings(w1402, "\r", w1393, " Offs(pStart,", w1399, w1390, w1398, w1390, w1397, ")" ("string"), w1390, w1396, w1390, w1391, w1390, w1389, ";" ("string"), w1388) -> (w1395:string)
                  }
                  frame True {
                  }
                }
              }
              frame True {
                n308 = case shown="False" w1414 {
                  tunnel: w1416 -> [w1437 w1438]
                  tunnel: w1409 -> [w1434 _]
                  tunnel: w1410 -> [w1433 _]
                  tunnel: w1408 -> [w1432 _]
                  tunnel: w1411 -> [w1431 _]
                  tunnel: [w1430 w1438] -> w1415
                  tunnel: w1413 -> [w1428 _]
                  tunnel: w1412 -> [w1426 _]
                  tunnel: w1407 -> [w1423 _]
                  tunnel: w1406 -> [w1422 _]
                  tunnel: w1405 -> [w1421 _]
                  tunnel: w1404 -> [w1420 _]
                  frame False {
                    w1425 = ","
                    n309 = local read "SET_tool"() -> (w1424:string)
                    n310 = Concatenate Strings(w1437, "\r", w1428, " RelTool(pStart,", w1434, w1425, w1433, w1425, w1432, "\\Rx:=" ("string"), w1422, "\\Ry:=" ("string"), w1421, "\\Rz:=" ("string"), w1420, ")" ("string"), w1425, w1431, w1425, w1426, w1425, w1424, ";" ("string"), w1423) -> (w1430:string)
                  }
                  frame True {
                  }
                }
              }
            }
            n311 = Empty String/Path?(string/path=w1371) -> (empty?=w1362:bool)
            n312 = Fract/Exp String To Number(use system decimal point (T)=FALSE ("Systemdezimalzeichen verwenden (T)"), string=w1282) -> (number=w1281:dbl)  [unwired: 2 in, 1 out]
          }
          n313 = local read "SET_term_moc"() -> (w1184:u16)
          n314 = case shown="1" w1184 {
            tunnel: ["" w1207 w1216 w1230 w1244] -> w1181
            tunnel: w1182 -> [_ w1206 w1217 w1231 w1245]
            tunnel: w1183 -> [_ w1201 w1215 w1229 w1243]
            frame 0, Default {
            }
            frame 1 {
              (unwired) FALSE ("Systemdezimalzeichen verwenden (T)")
              (unwired) i16 3 ("Genauigkeit (6)")
              w1208 = "\n\n        ! dont stop inside the model\n        MoveL Offs(pStart,50.0,50.0,"  # ! dont stop inside the model         MoveL Offs(pStart,50.0,50.0,
              n315 = local read "SET_term_z_offs"() -> (w1212:dbl)
              n316 = local read "SET_zone"() -> (w1213:i32)
              n317 = Add(x=w1212, y=w1201) -> (x+y=w1210:dbl)
              n318 = local read "SET_tool"() -> (w1214:string)
              n319 = Number To Decimal String(number=w1213) -> (decimal integer string=w1209:string)  [unwired: 1 in]
              n320 = Number To Fractional String(number=w1210) -> (F-format string=w1211:string)  [unwired: 3 in]
              n321 = Concatenate Strings(w1208, w1211, "),", w1206, ",z", w1209, "," ("String"), w1214, ";" ("String")) -> (w1207:string)
            }
            frame 2 {
              (unwired) FALSE ("Systemdezimalzeichen verwenden (T)")
              (unwired) i16 3 ("Genauigkeit (6)")
              w1222 = "\n\n        ! dont stop inside the model\n        MoveL Offs(pStart,-50.0,0.0,"  # ! dont stop inside the model         MoveL Offs(pStart,-50.0,0.0,
              n322 = local read "SET_term_z_offs"() -> (w1226:dbl)
              n323 = local read "SET_zone"() -> (w1227:i32)
              n324 = Add(x=w1226, y=w1215) -> (x+y=w1224:dbl)
              n325 = local read "SET_tool"() -> (w1228:string)
              n326 = Number To Decimal String(number=w1227) -> (decimal integer string=w1223:string)  [unwired: 1 in]
              n327 = Number To Fractional String(number=w1224) -> (F-format string=w1225:string)  [unwired: 3 in]
              n328 = Concatenate Strings(w1222, w1225, "),", w1217, ",z", w1223, "," ("String"), w1228, ";" ("String")) -> (w1216:string)
            }
            frame 3 {
              (unwired) FALSE ("Systemdezimalzeichen verwenden (T)")
              (unwired) i16 3 ("Genauigkeit (6)")
              w1236 = "\n\n        ! dont stop inside the model\n        MoveL Offs(pStart,0,-50.0,"  # ! dont stop inside the model         MoveL Offs(pStart,0,-50.0,
              n329 = local read "SET_term_z_offs"() -> (w1240:dbl)
              n330 = local read "SET_zone"() -> (w1241:i32)
              n331 = Add(x=w1240, y=w1229) -> (x+y=w1238:dbl)
              n332 = local read "SET_tool"() -> (w1242:string)
              n333 = Number To Decimal String(number=w1241) -> (decimal integer string=w1237:string)  [unwired: 1 in]
              n334 = Number To Fractional String(number=w1238) -> (F-format string=w1239:string)  [unwired: 3 in]
              n335 = Concatenate Strings(w1236, w1239, "),", w1231, ",z", w1237, "," ("String"), w1242, ";" ("String")) -> (w1230:string)
            }
            frame 4 {
              (unwired) FALSE ("Systemdezimalzeichen verwenden (T)")
              (unwired) i16 3 ("Genauigkeit (6)")
              w1250 = "\n\n        ! dont stop inside the model\n        MoveL Offs(pStart,0,0,"  # ! dont stop inside the model         MoveL Offs(pStart,0,0,
              n336 = local read "SET_term_z_offs"() -> (w1254:dbl)
              n337 = local read "SET_zone"() -> (w1255:i32)
              n338 = Add(x=w1254, y=w1243) -> (x+y=w1252:dbl)
              n339 = local read "SET_tool"() -> (w1256:string)
              n340 = Number To Decimal String(number=w1255) -> (decimal integer string=w1251:string)  [unwired: 1 in]
              n341 = Number To Fractional String(number=w1252) -> (F-format string=w1253:string)  [unwired: 3 in]
              n342 = Concatenate Strings(w1250, w1253, "),", w1245, ",z", w1251, "," ("String"), w1256, ";" ("String")) -> (w1244:string)
            }
          }
          n343 = Not(x=w1195) -> (.not. x?=w1194:bool)
          n344 = local write "CONV_running"(w1194) -> ()
          n345 = Concatenate Strings(w1196, w1181, w1186) -> (w1197:string)
        }
        frame True {
          w2057 = "File is empty!" ("message")
          n346 = One Button Dialog(message=w2057, button name ("OK")="End program") -> ()  [unwired: 1 out]
        }
      }
      n347 = Build Path(base path=w1140, name or relative path=w1139) -> (appended path=w1132:path)
      n348 = Open/Create/Replace File(file path (use dialog)=w1132, error in=errorcluster {"status"=FALSE, "code"=0, "source"=""}, operation (0:open)=T1."create", access (0:read/write)=enum16{"read/write", "read-only", "write-only"}."read/write") -> (refnum out=w1129:refnum<file>, error out=w1130:errorcluster)  [unwired: 2 in, 1 out]
      n349 = Unbundle(w1130) -> ("status"=w1133:bool)  [unwired: 2 out]
      n350 = case shown="True" w1133 {
        tunnel: w1132 -> [_ w1158]
        tunnel: w1131 -> [w1152 w1157]
        tunnel: w1130 -> [w1153 _]
        tunnel: w1129 -> [w1151 _]
        frame False {
          n351 = Write to Text File(file (use dialog)=w1151, text=w1152, error in=w1153) -> (refnum out=w1154:refnum<file>, error out=w1155:errorcluster)  [unwired: 1 in, 1 out]
          n352 = local write "OUT_rapid"(w1152) -> ()
          n353 = Close File(refnum=w1154, error in=w1155) -> (error out=w1156:errorcluster)  [unwired: 1 out]
          n354 = local write "ERR_write_file"(w1156) -> ()
        }
        frame True {
          n355 = flat-sequence {
            tunnel: w1158 -> [w1167]
            tunnel: w1157 -> [w1168]
            frame #0 {
              n356 = Two Button Dialog(message="CAUTION!\n\nFile with the same name\nalready exists. Do you want to\noverwrite?", 1:"EXIT PROGRAM" ("F button name (\"Cancel\")"), 2:"OVERWRITE" ("T button name (\"OK\")")) -> (T button?=w1159:bool)
              n357 = Not(x=w1159) -> (.not. x?=w1160:bool)
              n358 = Stop(stop? (T)=w1160) -> ()
            }
            frame #1 {
              n359 = Open/Create/Replace File(file path (use dialog)=w1167, error in=errorcluster {"status"=FALSE, "code"=0, "source"=""}, operation (0:open)=T1."replace or create", access (0:read/write)=enum16{"read/write", "read-only", "write-only"}."read/write") -> (refnum out=w1166:refnum<file>, error out=w1165:errorcluster)  [unwired: 2 in, 1 out]
              n360 = Write to Text File(file (use dialog)=w1166, text=w1168, error in=w1165) -> (refnum out=w1169:refnum<file>, error out=w1170:errorcluster)  [unwired: 1 in, 1 out]
              n361 = local write "OUT_rapid"(w1168) -> ()
              n362 = Close File(refnum=w1169, error in=w1170) -> (error out=w1171:errorcluster)  [unwired: 1 out]
              n363 = local write "ERR_write_file"(w1171) -> ()
            }
          }
        }
      }
    }
  }
